vi "Get MCC AI DAQ Data.vi"(8 "error in (no error)":errorcluster, 10 "Phase":T2, 11 "DAQ_Engine in":refnum<class "DAQ_Engine.lvclass">) -> (0 "error out":errorcluster, 1 "Start time":timestamp, 2 "Data[]":dbl[](array[numeric]), 3 "DAQ_Engine out":refnum<class "DAQ_Engine.lvclass">, 4 "error":bool, 5 "DataCnt":i32, 7 "MeasSettings*":T1={"Data Rate 9775"=3.0, "Data Rate 9215"=1200000.0, "Samples RMS 9215"=480000, "Samples RMS 9775"=3})   [LabVIEW 2019, in "DAQ_Engine.lvclass"]
doc: "Developed by Kevin Thompson\nkevin@thompsonengineering.net\n\nCopyright 2020\nThompson Engineering, LLC"
uses:
  DAQ_Engine.lvclass
  support/DAQ Lib/ToEng(array).vi
  Common/DataTypes/Phase Selection--enum.ctl
  Common/DataTypes/Measurement Config--cluster.ctl
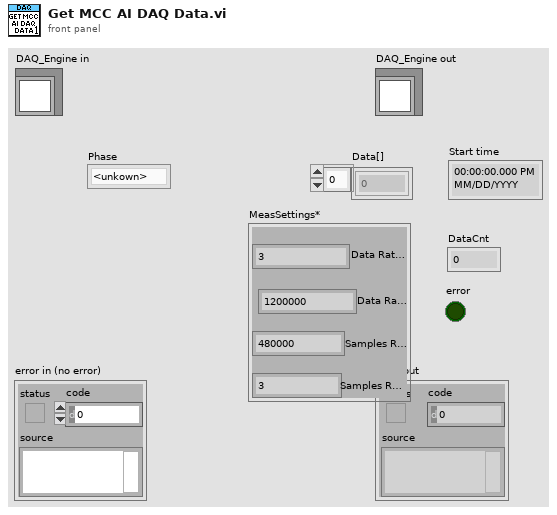
[diagram p1: front panel]
types:
  T1 = typedef "Measurement Config--cluster.ctl" = cluster{"Data Rate 9775":dbl, "Data Rate 9215":dbl, "Samples RMS 9215":u32, "Samples RMS 9775":u32}
  T2 = typedef "Phase Selection--enum.ctl" = enum16{"<unkown>", "Phase 1", "Phase 2", "Phase 3", "Single"}
  T3 = typedef "DAQ_Engine.lvclass/Settings--cluster.ctl" = cluster{"Simulation":bool, "Initial ErrReporting setting":i32, "Initial Measurement settings":T1, "BoardNum":T4, "Acquisition mode":T5, "DemoMode":bool}
  T4 = typedef "DAQ_Engine.lvclass/BoardNum--cluster.ctl" = cluster{"P1Sgl":u32, "P2":u32, "P3":u32}
  T5 = typedef "Acquisition Mode--cluster.ctl" = enum16{"3phase", "Single"}
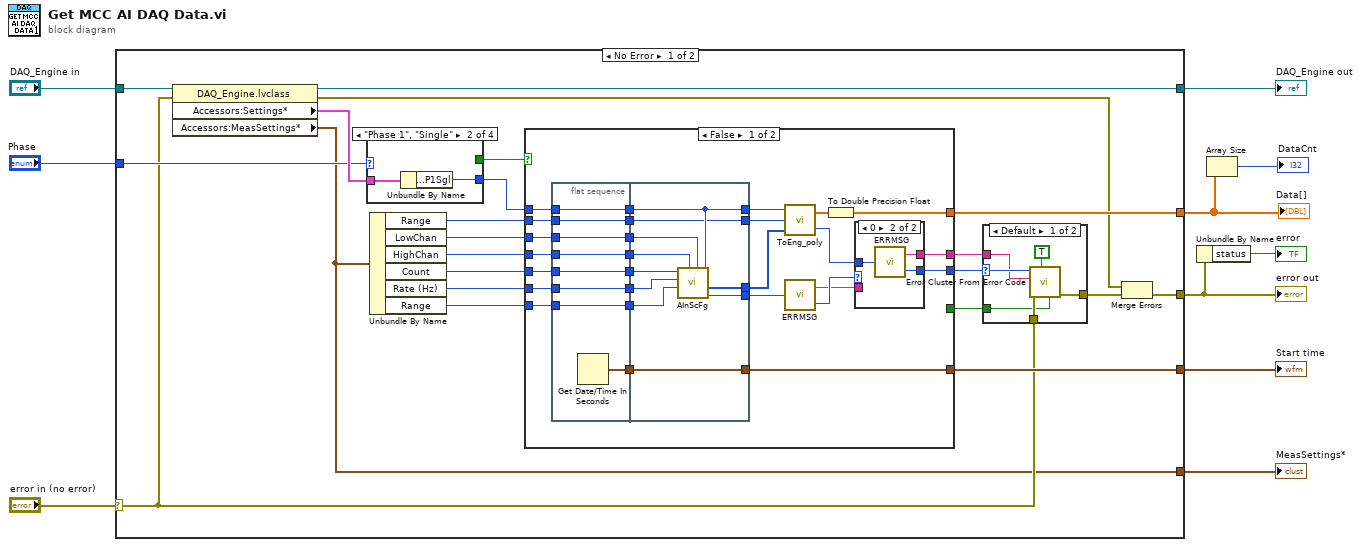
[diagram p0: block diagram]
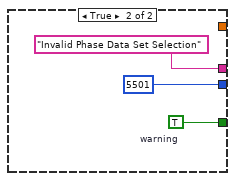
[diagram p3: hidden frame]
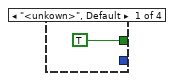
[diagram p5: hidden frame]
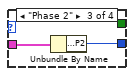
[diagram p6: hidden frame]
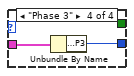
[diagram p7: hidden frame]
diagram:
  n1 = case shown="No Error" "error in (no error)" {
    selector: "error in (no error)" -> [w15 w101]
    tunnel: [w14 w101] -> w5
    tunnel: [w27 w100] -> w8
    tunnel: "DAQ_Engine in" -> [w31 w100]
    tunnel: [w30 _] -> w7
    tunnel: "Phase" -> [w28 _]
    tunnel: [w19 _] -> w3
    tunnel: [w12 _] -> w1
    frame No Error {
      n2 = property class="DAQ_Engine.lvclass"(reference=w31, error in=w15) -> (reference out=w27:refnum<class "DAQ_Engine.lvclass">, error out=w13:errorcluster, "Accessors:Settings*"=w29:T3, "Accessors:MeasSettings*"=w12:T1)
      n3 = case shown="\"Phase 1\", \"Single\"" w28 {
        tunnel: w29 -> [_ w95 w97 w99]
        tunnel: [_ w94 w96 w98] -> w22
        tunnel: [TRUE _ _ _] -> w18
        frame "<unkown>", Default {
        }
        frame "Phase 1", "Single" {
          n4 = Unbundle By Name(w95) -> ("BoardNum.P1Sgl"=w94:u32)
        }
        frame "Phase 2" {
          n5 = Unbundle By Name(w97) -> ("BoardNum.P2"=w96:u32)
        }
        frame "Phase 3" {
          n6 = Unbundle By Name(w99) -> ("BoardNum.P3"=w98:u32)
        }
      }
      n7 = Unbundle By Name(w12) -> ("Range"=w21:i32, "LowChan"=w23:i32, "HighChan"=w32:i32, "Count"=w24:i32, "Rate (Hz)"=w25:i32, "Range"=w26:i32)
      n8 = case shown="False" w18 {
        tunnel: w32 -> [w51 _]
        tunnel: [w49 _] -> w30
        tunnel: w26 -> [w48 _]
        tunnel: w25 -> [w47 _]
        tunnel: w24 -> [w46 _]
        tunnel: w23 -> [w45 _]
        tunnel: w22 -> [w43 _]
        tunnel: w21 -> [w41 _]
        tunnel: [w33 _] -> w19
        tunnel: [w35 5501 ("ErrCode (Out)")] -> w17
        tunnel: [w34 "Invalid Phase Data Set Selection" ("ErrMsg")] -> w16
        tunnel: [_ w83] -> w11
        frame False {
          n9 = flat-sequence {
            tunnel: w51 -> [w72]
            tunnel: [w72] -> w59
            tunnel: [w71] -> w58
            tunnel: w48 -> [w70]
            tunnel: [w70] -> w57
            tunnel: w47 -> [w69]
            tunnel: [w69] -> w56
            tunnel: w46 -> [w68]
            tunnel: [w68] -> w55
            tunnel: w45 -> [w67]
            tunnel: [w67] -> w54
            tunnel: [w66] -> w53
            tunnel: w43 -> [w66]
            tunnel: [w65] -> w52
            tunnel: w41 -> [w65]
            tunnel: [w82] -> w50
            tunnel: [w80] -> w44
            tunnel: w59 -> [w81]
            tunnel: [w79] -> w49
            tunnel: w58 -> [w79]
            tunnel: w57 -> [w78]
            tunnel: w56 -> [w77]
            tunnel: w55 -> [w76]
            tunnel: w54 -> [w75]
            tunnel: w53 -> [w74]
            tunnel: [w74] -> w42
            tunnel: [w73] -> w40
            tunnel: w52 -> [w73]
            frame #0 {
              n10 = Get Date/Time In Seconds() -> (seconds since 1Jan1904=w71:timestamp)
            }
            frame #1 {
              n11 = call "AInScFg.VI"("BoardNum"=w74, "LowChan"=w75, "HighChan"=w81, "Range"=w78, "Rate"=w77, "Count"=w76) -> ("ErrCode"=w82:i32, "ADData"=w80:u16[])  [unwired: 2 in, 1 out]
            }
          }
          n12 = call-poly "ToEng_poly.VI"("AD Data"=w44, "Range"=w40, "BoardNum"=w42) -> ("ErrCode"=w36:i32, "Eng Units"=w39:sgl[])
          n13 = call "ERRMSG.VI"("ErrCode"=w50) -> ("ErrMsg"=w37:string, "ErrCode (Out)"=w38:i32)
          n14 = To Double Precision Float(number=w39) -> (double precision float=w33:dbl[])
          n15 = case shown="0" w38 {
            selector: w38 -> [w61 _]
            tunnel: w36 -> [_ w64]
            tunnel: [w61 w63] -> w35
            tunnel: w37 -> [w60 _]
            tunnel: [w60 w62] -> w34
            frame Default {
            }
            frame 0 {
              n16 = call "ERRMSG.VI"("ErrCode"=w64) -> ("ErrMsg"=w62:string, "ErrCode (Out)"=w63:i32)
            }
          }
        }
        frame True {
          w83 = TRUE  # warning
        }
      }
      n17 = case shown="Default" w17 {
        selector: w17 -> [w90 _]
        tunnel: [w91 w92] -> w20
        tunnel: w16 -> [w89 _]
        tunnel: w15 -> [w88 w92]
        tunnel: w11 -> [w86 _]
        frame Default {
          n18 = call <vilib>:"Error Cluster From Error Code.vi"("is warning? (False)"=w86, "show call chain? (False)"=TRUE, "error in (no error)"=w88, "error message (\"\")"=w89, "error code (0)"=w90) -> ("error out"=w91:errorcluster)  [unwired: 4 in]
        }
        frame 0 {
        }
      }
      n19 = Merge Errors(w13, w20) -> (w14:errorcluster)
    }
    frame Error {
    }
  }
  "error out" <- w5
  "DAQ_Engine out" <- w8
  "Start time" <- w7
  "Data[]" <- w3
  "MeasSettings*" <- w1
  n20 = Unbundle By Name(w5) -> ("status"=→"error":bool)
  n21 = Array Size(array=w3) -> (size(s)=→"DataCnt":i32)
